vi "Write httpHeaders.vi"(8 "error in (no error)":errorcluster, 10 "Headers":refnum<class "httpHeaders.lvclass">, 11 "httpRequest in":refnum<class "httpRequest.lvclass">) -> (0 "error out":errorcluster, 3 "httpRequest out":refnum<class "httpRequest.lvclass">)   [LabVIEW 2020, in "httpClient.lvlib" / "httpRequest.lvclass"]
uses:
  httpRequest.lvclass
  httpHeaders/httpHeaders.lvclass
  httpRequest.lvclass/httpRequest.ctl
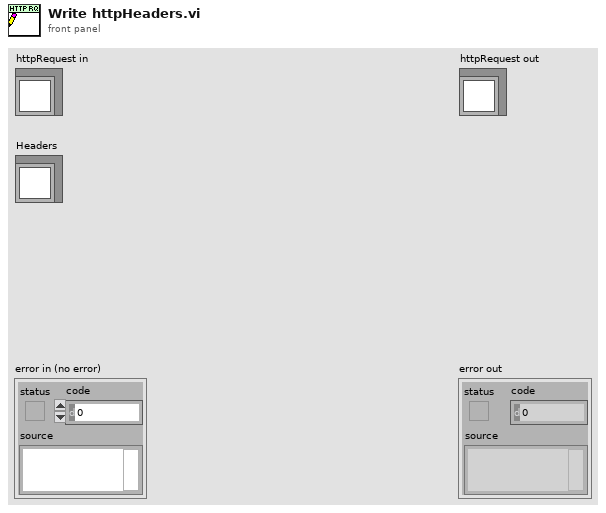
[diagram p1: front panel]
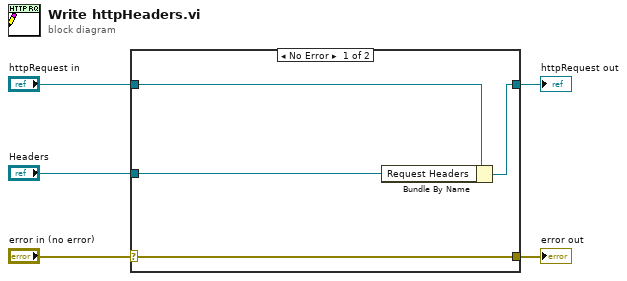
[diagram p0: block diagram]
diagram:
  n1 = case shown="No Error" "error in (no error)" {
    selector: "error in (no error)" -> [w9 w10]
    tunnel: [w9 w10] -> w4
    tunnel: [w7 w11] -> w2
    tunnel: "httpRequest in" -> [w8 w11]
    tunnel: "Headers" -> [w6 _]
    frame No Error {
      n2 = Bundle By Name(cluster=w8, "Request Headers"=w6) -> (w7:refnum<class "httpRequest.lvclass">)
    }
    frame Error {
    }
  }
  "error out" <- w4
  "httpRequest out" <- w2
